vi "Shuffle Array.vi"(5 "Point":T13, 6 "XRef":refnum<vi>, 7 "State In":T14) -> (0 "Subitem Help Info":T1, 1 "Detailed Help Info":T10, 2 "Standard Help Info":T8, 3 "Use Subitem Help?":bool, 4 "Use Detailed Help?":bool)   [LabVIEW 2018, in "Shuffle Array.xnode"]
doc: "Shuffles the elements of the input array into a random order. For 2D arrays can shuffle rows, columns or individual elements depending on the rank input."
uses:
  Shuffle Array.xnode
  State.ctl
  <vilib>/XNodeSupport/XNodePoint.ctl
  <vilib>/XNodeSupport/XNodeInt.ctl
  <vilib>/XNodeSupport/XNodeDetailedHelpInfo.ctl
  <vilib>/XNodeSupport/XNodeImage.ctl
  <vilib>/XNodeSupport/XNodeRect32.ctl
  <vilib>/XNodeSupport/XNodeTerms.ctl
  <vilib>/XNodeSupport/XNodeTerm.ctl
  <vilib>/XNodeSupport/XNodeString.ctl
  <vilib>/XNodeSupport/XNodeVariant.ctl
  <vilib>/XNodeSupport/XNodeBool.ctl
  <vilib>/XNodeSupport/XNodeStandardHelpInfo.ctl
  <vilib>/XNodeSupport/XNodePath.ctl
  <vilib>/XNodeSupport/XNodeSubitemHelpInfo.ctl
  <vilib>/XNodeSupport/NI_XNodeSupport.lvlib
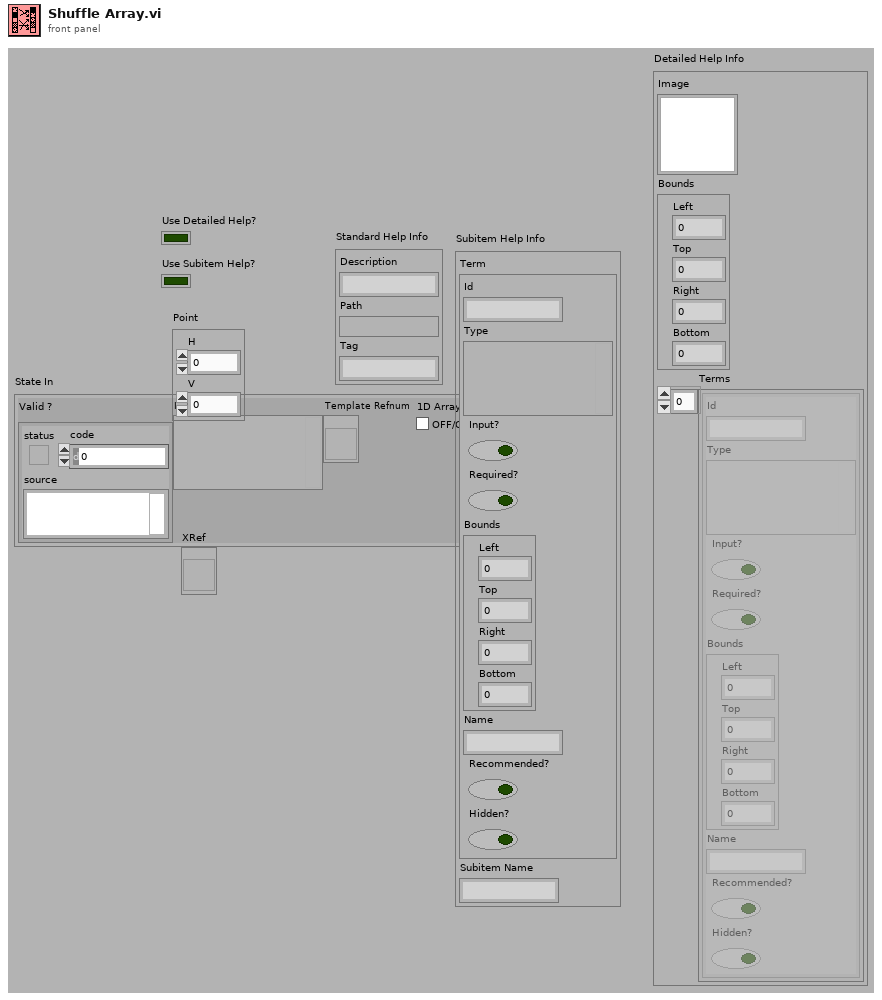
[diagram p1: front panel]
types:
  T1 = typedef "NI_XNodeSupport.lvlib/XNodeSubitemHelpInfo.ctl" = cluster{"Term":T2, "Subitem Name":T3}
  T2 = typedef "NI_XNodeSupport.lvlib/XNodeTerm.ctl" = cluster{"Id":T3, "Type":T4, "Input?":T5, "Required?":T5, "Bounds":T6, "Name":T3, "Recommended?":T5, "Hidden?":T5}
  T3 = typedef "NI_XNodeSupport.lvlib/XNodeString.ctl" = string
  T4 = typedef "NI_XNodeSupport.lvlib/XNodeVariant.ctl" = variant
  T5 = typedef "NI_XNodeSupport.lvlib/XNodeBool.ctl" = bool
  T6 = typedef "NI_XNodeSupport.lvlib/XNodeRect32.ctl" = cluster{"Left":T7, "Top":T7, "Right":T7, "Bottom":T7}
  T7 = typedef "NI_XNodeSupport.lvlib/XNodeInt.ctl" = i32
  T8 = typedef "NI_XNodeSupport.lvlib/XNodeStandardHelpInfo.ctl" = cluster{"Description":T3, "Path":T9, "Tag":T3}
  T9 = typedef "NI_XNodeSupport.lvlib/XNodePath.ctl" = path
  T10 = typedef "NI_XNodeSupport.lvlib/XNodeDetailedHelpInfo.ctl" = cluster{"Image":T11, "Bounds":T6, "Terms":T12}
  T11 = typedef "NI_XNodeSupport.lvlib/XNodeImage.ctl" = picture
  T12 = typedef "NI_XNodeSupport.lvlib/XNodeTerms.ctl" = T2[]
  T13 = typedef "NI_XNodeSupport.lvlib/XNodePoint.ctl" = cluster{"H":T7, "V":T7}
  T14 = typedef "Shuffle Array.xnode/State.ctl" = cluster{"Valid ?":errorcluster, "Input Type":variant, "Template Refnum":refnum<vi>, "1D Array ?":bool}
  T15 = typedef "NI_XNodeSupport.lvlib/XNodeTerm3Array.ctl" = T16[]
  T16 = typedef "NI_XNodeSupport.lvlib/XNodeTerm3.ctl" = cluster{"Name":T3, "Id":T3, "Type":T4, "Bounds":T6, "Input?":T5, "Required?":T5, "Recommended?":T5, "Adaptive?":T5, "Hidden?":T5, "Direction":T17, "Break Wire?":T5}
  T17 = typedef "NI_XNodeSupport.lvlib/XNodeTermDirection.ctl" = enum32{"Auto", "Up", "Down", "Left", "Right", "Center"}
  T18 = cluster{"Description":string, "Help.Path":path, "Help.Tag":string}
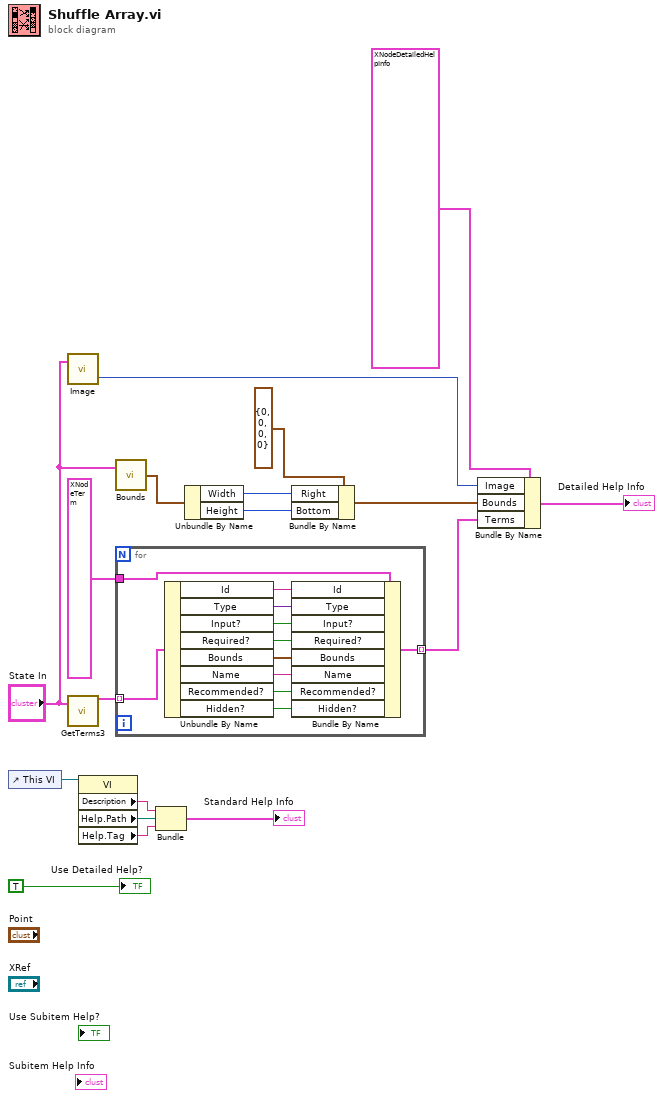
[diagram p0: block diagram]
diagram:
  n1 = control-ref of="This VI"() -> (w6:refnum<vi>)
  n2 = call "Image.vi"("State In"="State In") -> ("Image"=w13:picture)  [unwired: 1 in, 1 out]
  n3 = call "GetTerms3.vi"("State In"="State In") -> ("Terms"=w17:T15)  [unwired: 1 in, 17 out]
  n4 = property class="VI"(reference=w6) -> ("Description"=w5:string, "Help.Path"=w4:path, "Help.Tag"=w3:string)  [unwired: 1 in, 2 out]
  n5 = call "Bounds.vi"("State In"="State In") -> ("Bounds"=w10:cluster{"Width":T7, "Height":T7})  [unwired: 1 in]
  n6 = for {
    tunnel: T2 {"Id"="", "Type"=variant, "Input?"=FALSE, "Required?"=FALSE, "Bounds"={"Left"=0, "Top"=0, "Right"=0, "Bottom"=0}, "Name"="", "Recommended?"=FALSE, "Hidden?"=FALSE} ("Term") -> [w29]
    tunnel: w17 -> [w28] mode=indexing
    tunnel: [w19] -> w15 mode=indexing
    n7 = Unbundle By Name(w28) -> ("Id"=w27:T3, "Type"=w26:T4, "Input?"=w25:T5, "Required?"=w24:T5, "Bounds"=w23:T6, "Name"=w22:T3, "Recommended?"=w21:T5, "Hidden?"=w20:T5)
    n8 = Bundle By Name(cluster=w29, "Id"=w27, "Type"=w26, "Input?"=w25, "Required?"=w24, "Bounds"=w23, "Name"=w22, "Recommended?"=w21, "Hidden?"=w20) -> (w19:T2)
  }
  n9 = Bundle("Description"=w5, "Help.Path"=w4, "Help.Tag"=w3) -> (→"Standard Help Info":T18)  [unwired: 1 out]
  n10 = Unbundle By Name(w10) -> ("Width"=w9:T7, "Height"=w8:T7)
  n11 = Bundle By Name(cluster=T6 {"Left"=0, "Top"=0, "Right"=0, "Bottom"=0} ("Bounds"), "Right"=w9, "Bottom"=w8) -> (w7:T6)
  n12 = Bundle By Name(cluster=T10 {"Image"=bytes[0], "Bounds"={"Left"=0, "Top"=0, "Right"=0, "Bottom"=0}, "Terms"=[]} ("Detailed Help Info"), "Image"=w13, "Bounds"=w7, "Terms"=w15) -> (→"Detailed Help Info":T10)
  "Use Detailed Help?" <- TRUE ("Use Detailed Help?")
